vi "Atof.vi"(7 "string":string) -> (3 "number":dbl=nan)   [LabVIEW 2020]
doc: "Converts a string to a double precision floating point number.\n\nSpecial strings such as \"NaN, \"+Inf\", \"Inf\", and \"-Inf\" are converted appropriately. Scientific notation is not recognized. An empty string (after filtering) is converted to \"NaN\". \n\nWhitespace is trimmed and all characters are converted to uppercase before the conversion. If \"NaN, \"+Inf\", \"Inf\", or \"-Inf\" are found, they are converted appropriately. Otherwise, all characters except: 0-9, plus, minus, and decimal point are removed. The remaining characters are converted to a floating point number or \"NaN\"."
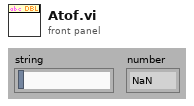
[diagram p1: front panel]
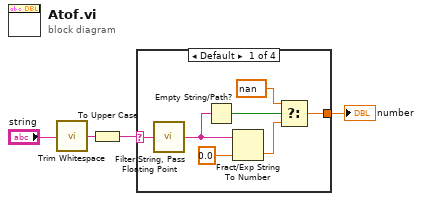
[diagram p0: block diagram]
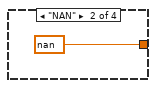
[diagram p2: hidden frame]
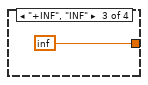
[diagram p3: hidden frame]
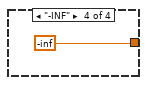
[diagram p4: hidden frame]
diagram:
  n1 = call <vilib>:"Trim Whitespace.vi"("string"="string") -> ("trimmed string"=w2:string)  [unwired: 1 in]
  n2 = To Upper Case(1:w2) -> (0:w1:string)
  n3 = case shown="Default" w1 {
    selector: w1 -> [w10 _ _ _]
    tunnel: [w5 nan ("t") inf -inf] -> w4
    frame Default {
      n4 = call "Filter String, Pass Floating Point.vi"("Input String"=w10) -> ("Numeric String"=w9:string)
      n5 = Empty String/Path?(string/path=w9) -> (empty?=w8:bool)
      n6 = Fract/Exp String To Number(string=w9, default (0 dbl)=0.0 ("Result")) -> (number=w7:dbl)  [unwired: 2 in, 1 out]
      n7 = Select(t=nan, s=w8, f=w7) -> (s? t:f=w5:dbl)
    }
    frame "NAN" {
    }
    frame "+INF", "INF" {
    }
    frame "-INF" {
    }
  }
  "number" <- w4
